vi "Squeezing Triggered Phase Extraction.vi"(0 "Input Data":dbl[](array[numeric]), 1 "sampling freq: fs":dbl=5000000.0, 5 "low cutoff freq: fl":dbl=200.0, 7 "Measurement indices":dbl[](array[numeric]), 9 "order":i32=2, 11 "dt":dbl=2e-07, 12 "sampling info":cluster{"Fs":dbl, "#s":dbl}={"Fs"=5000000.0, "#s"=130000.0}) -> (3 "Envelope":dbl[](graph), 4 "detected frequency":dbl format="%.4p", 6 "detected phase (deg)":dbl format="%.2p", 8 "Squeezing Arches Phase Array":dbl[](graph), 10 "Phase Array of Squeezed Pulses":dbl[](graph), 14 "Normalized Envelope":waveform(dbl)(graph))   [LabVIEW 2009]
uses:
  <vilib>/measure/matone.llb/Extract Single Tone Information 1 Chan.vi
  <vilib>/Analysis/3filter.llb/Butterworth Filter (DBL).vi
  <vilib>/Analysis/NI_AALBase.lvlib
  <vilib>/measure/NI_MAPro.lvlib
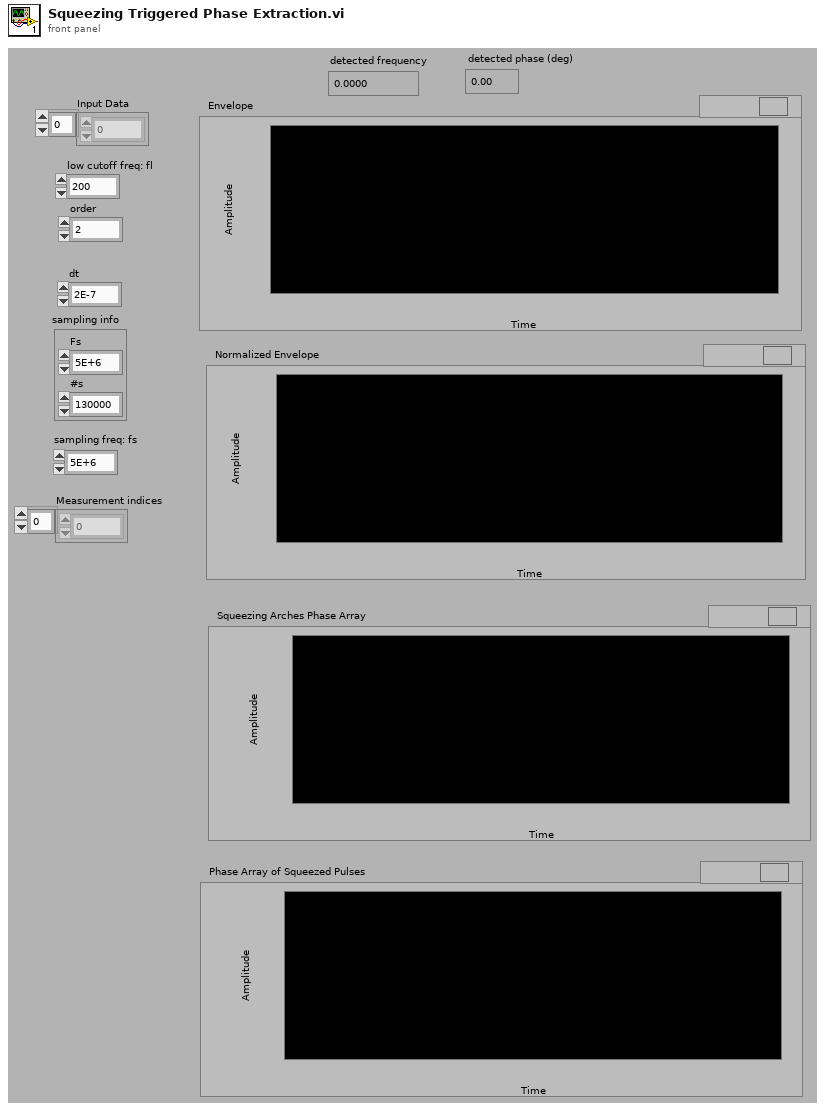
[diagram p1: front panel]
types:
  T1 = enum32{"Lowpass", "Highpass", "Bandpass", "Bandstop"}
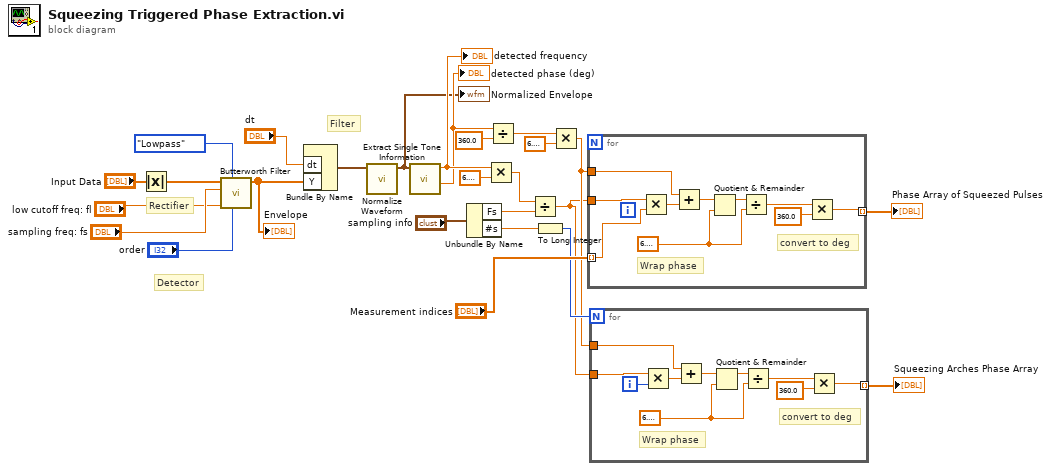
[diagram p0: block diagram]
diagram:
  # "Detector"
  # "Filter"
  # "Rectifier"
  n1 = Absolute Value(x="Input Data") -> (abs(x)=w7:dbl[])
  n2 = call-poly <vilib>:"Butterworth Filter.vi"("order"="order", "filter type"=T1."Lowpass", "low cutoff freq: fl"="low cutoff freq: fl", "sampling freq: fs"="sampling freq: fs", "X"=w7) -> ("Filtered X"=w24:dbl[])  [unwired: 3 in, 1 out]
  "Envelope" <- w24
  n3 = Bundle By Name("dt"="dt", "Y"=w24) -> (w12:waveform(dbl))  [unwired: 1 in]
  n4 = call <vilib>:"Normalize Waveform.vi"("waveform in"=w12) -> ("normalized waveform"=w13:waveform(dbl))  [unwired: 7 in, 3 out]
  "Normalized Envelope" <- w13
  n5 = call-poly <vilib>:"Extract Single Tone Information.vi"("time signal in"=w13) -> ("detected phase (deg)"=w22:dbl, "detected frequency"=w23:dbl)  [unwired: 5 in, 4 out]
  "detected frequency" <- w23
  "detected phase (deg)" <- w22
  n6 = Unbundle By Name("sampling info") -> ("Fs"=w15:dbl, "#s"=w14:dbl)
  n7 = Multiply(x=w23, y=6.283185307179586) -> (x*y=w16:dbl)
  n8 = Divide(x=w22, y=360.0) -> (x/y=w19:dbl)
  n9 = Divide(x=w16, y=w15) -> (x/y=w1:dbl)
  n10 = To Long Integer(number=w14) -> (32bit integer=w3:i32)
  n11 = Multiply(x=w19, y=6.283185307179586) -> (x*y=w2:dbl)
  n12 = for {
    tunnel: w1 -> [w36]
    tunnel: w2 -> [w35]
    tunnel: [w30] -> w26 mode=indexing
    tunnel: "Measurement indices" -> [w27] mode=indexing
    w33 = 6.283185307179586
    # "convert to deg"
    # "Wrap phase"
    n13 = Multiply(x=w36, y=w27) -> (x*y=w34:dbl)
    n14 = Add(x=w35, y=w34) -> (x+y=w29:dbl)
    n15 = Quotient & Remainder(x=w29, y=w33) -> (x-y*floor(x/y)=w28:dbl)  [unwired: 1 out]
    n16 = Divide(x=w28, y=w33) -> (x/y=w32:dbl)
    n17 = Multiply(x=w32, y=360.0) -> (x*y=w30:dbl)
  }
  "Phase Array of Squeezed Pulses" <- w26
  n18 = for {
    N: w3 -> [_]
    tunnel: w1 -> [w46]
    tunnel: w2 -> [w45]
    tunnel: [w40] -> w4 mode=indexing
    i -> [w37]
    w43 = 6.283185307179586
    # "convert to deg"
    # "Wrap phase"
    n19 = Multiply(x=w46, y=w37) -> (x*y=w44:dbl)
    n20 = Add(x=w45, y=w44) -> (x+y=w39:dbl)
    n21 = Quotient & Remainder(x=w39, y=w43) -> (x-y*floor(x/y)=w38:dbl)  [unwired: 1 out]
    n22 = Divide(x=w38, y=w43) -> (x/y=w42:dbl)
    n23 = Multiply(x=w42, y=360.0) -> (x*y=w40:dbl)
  }
  "Squeezing Arches Phase Array" <- w4
